vi "tcp_get_data.vi"(8 "error in":errorcluster, 10 "devs_info":T1[](array[typedef]), 11 "TCP Network Connection in":refnum<k5>) -> (0 "error out":errorcluster, 2 "data_out":u8[][](array[numeric]), 3 "TCP Network Connection out":refnum<k5>)   [LabVIEW 2021]
uses:
  typedefs/dev_full_info.ctl
  typedefs/dev_states.ctl
  typedefs/send_states.ctl
  typedefs/w5500_cmd.ctl
  typedefs/w5500_pck.ctl
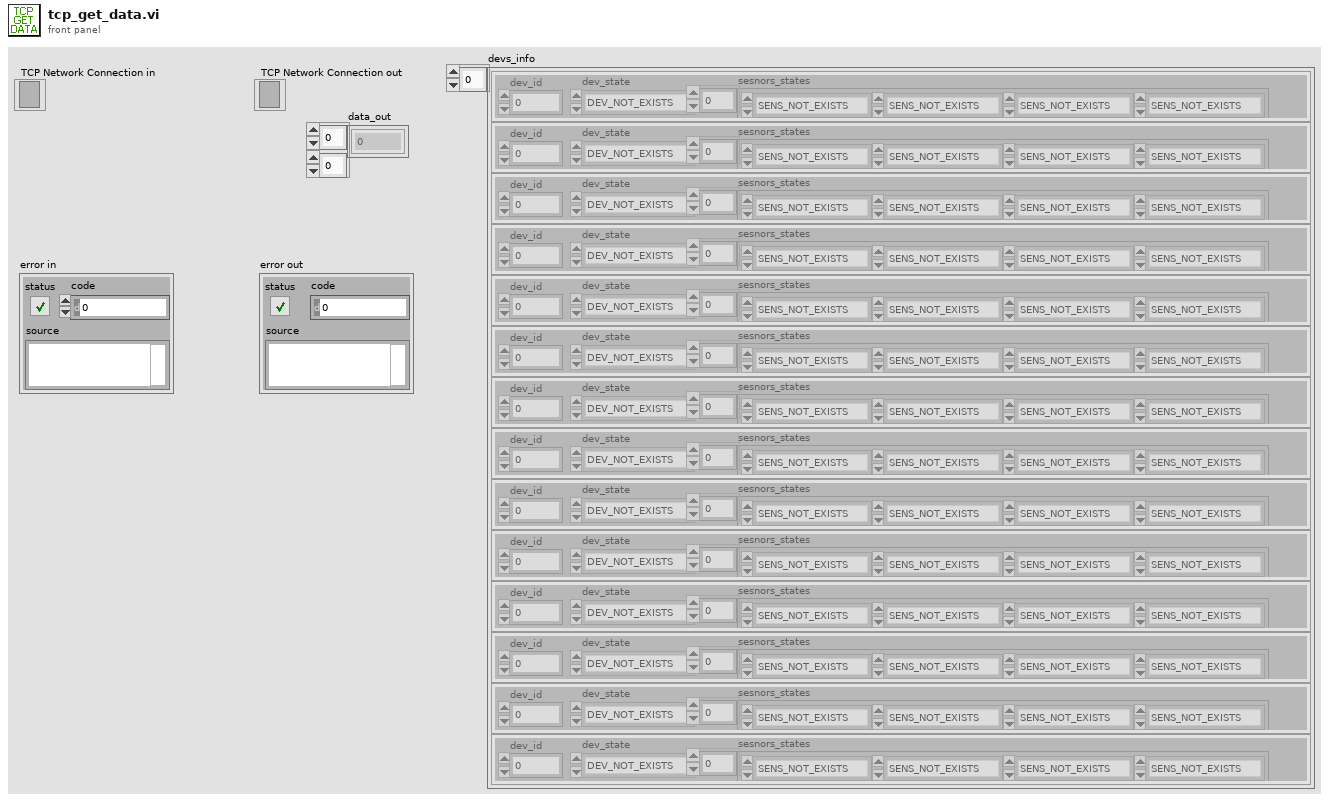
[diagram p1: front panel]
types:
  T1 = typedef "dev_full_info.ctl" = cluster{"dev_id":u32, "dev_state":T2, "sesnors_states":T3[]}
  T2 = typedef "dev_states.ctl" = enum16{"DEV_NOT_EXISTS", "DEV_EXISTS", "DEV_ERROR", "DEV_CRC_ERROR"}
  T3 = typedef "send_states.ctl" = enum16{"SENS_NOT_EXISTS", "SENS_EXISTS"}
  T4 = typedef "w5500_pck.ctl" = cluster{"cmd_type":T5, "pck_num":u32, "dev_id":u32, "data":u8[]}
  T5 = typedef "w5500_cmd.ctl" = enum32{"LAN_TRANS_START", "LAN_DATA_SZ", "LAN_CHUNK_SEND", "LAN_CHUNK_ACK", "LAN_DEVS_INFO", "LAN_DEVS_NUM", "LAN_DEVS_EXS", "LAN_DEVS_ACK", "LAN_CMD_ACK", "LAN_CMD_FIN", "LAN_SND_STAT", "LAN_REQ_STAT", "LAN_ANS_STAT", "LAN_ERR_STAT", "LAN_SETT_SET", "LAN_SETT_GET", "LAN_SETT_ACK", "LAN_SETT_ERR"}
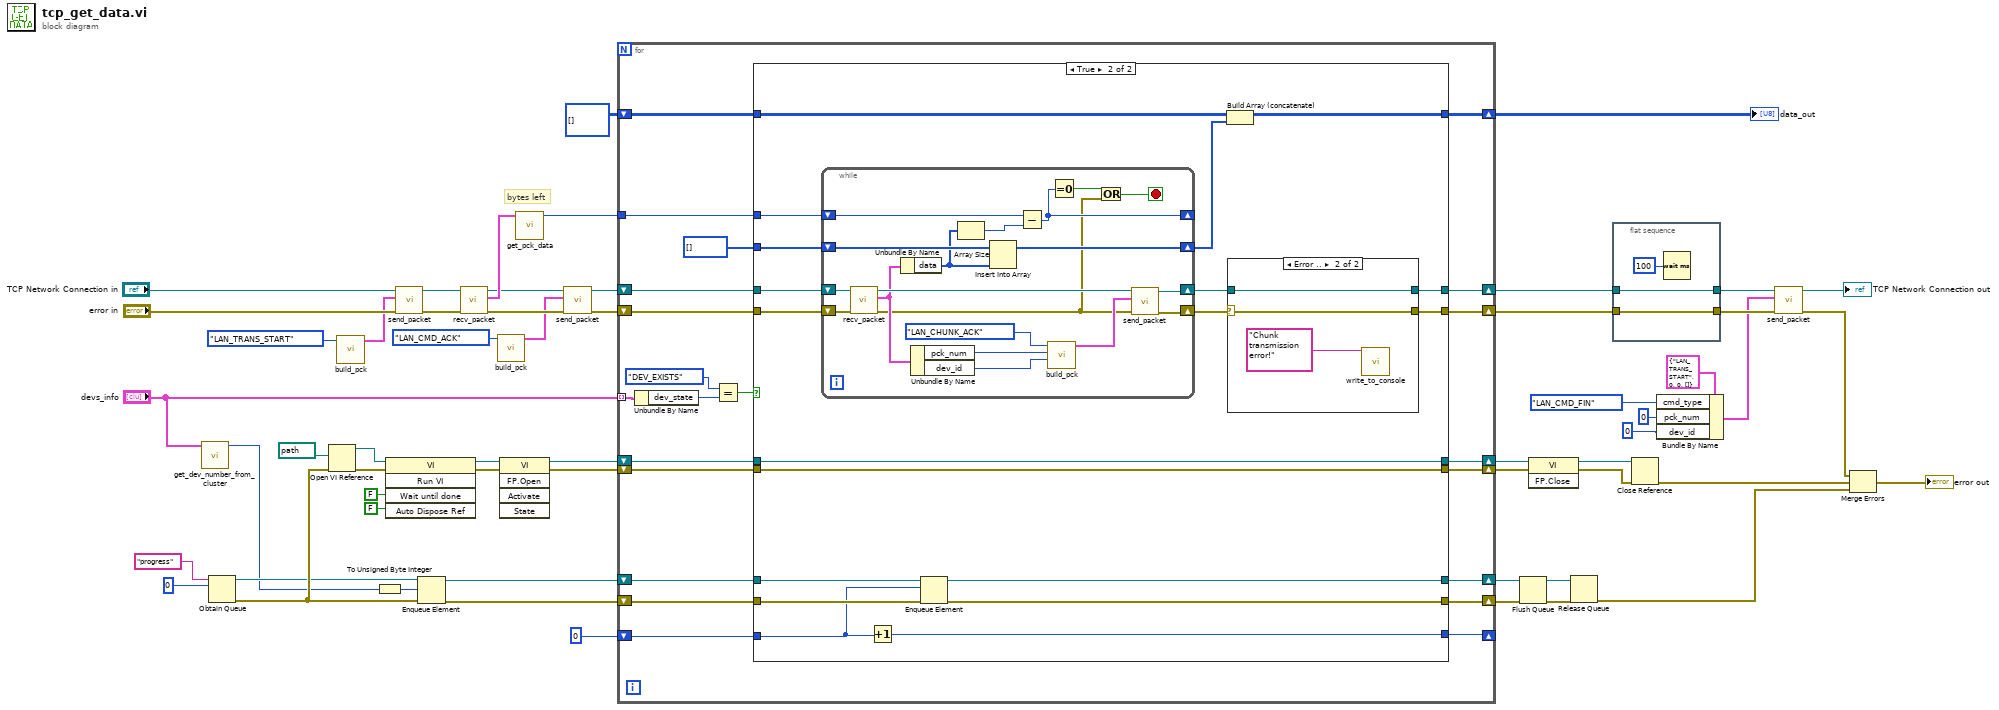
[diagram p0: block diagram]
diagram:
  # "bytes left"
  n1 = call "get_dev_number_from_cluster.vi"("devs_info"="devs_info") -> ("dev_num"=w13:u16)  [unwired: 10 in]
  n2 = Obtain Queue(name (unnamed)="progress", element data type=u8 0) -> (queue out=w20:refnum<queue>, error out=w21:errorcluster)  [unwired: 3 in, 1 out]
  n3 = Open VI Reference(vi path=path "C:/Users/Mi/YandexDisk/BigProjects/Линейки Холлов/lv2021/Users/Mi/YandexDisk/BigProjects/Линейки Холлов/labview/utils/progress_bar.vi", error in (no error)=w21) -> (vi reference=w29:refnum<vi>, error out=w28:errorcluster)  [unwired: 4 in]
  n4 = call "build_pck.vi"("cmd_type"=w5500_cmd."LAN_TRANS_START") -> ("w5500_pck"=w45:T4)  [unwired: 10 in]
  n5 = To Unsigned Byte Integer(number=w13) -> (unsigned 8bit integer=w14:u8)
  n6 = invoke class="VI" method="Run VI"(reference=w29, error in=w28, "Wait until done"=FALSE ("Wait Until Done"), "Auto Dispose Ref"=FALSE ("Auto Dispose Reference")) -> (reference out=w22:refnum<vi>, error out=w23:errorcluster)  [unwired: 1 in, 3 out]
  n7 = call "send_packet.vi"("error in (no error)"="error in", "w5500_pck in"=w45, "TCP Network Connection in"="TCP Network Connection in") -> ("error out"=w53:errorcluster, "TCP Network Connection out"=w54:refnum<k5>)  [unwired: 7 in]
  n8 = Enqueue Element(queue=w20, element=w14, error in (no error)=w21) -> (queue out=w16:refnum<queue>, error out=w17:errorcluster)  [unwired: 1 in, 1 out]
  n9 = call "recv_packet.vi"("error in (no error)"=w53, "TCP Network Connection in"=w54) -> ("error out"=w41:errorcluster, "w5500_pck"=w46:T4, "TCP Network Connection out"=w42:refnum<k5>)  [unwired: 7 in]
  n10 = call "build_pck.vi"("cmd_type"=w5500_cmd."LAN_CMD_ACK") -> ("w5500_pck"=w37:T4)  [unwired: 10 in]
  n11 = invoke class="VI" method="FP.Open"(reference=w22, error in=w23) -> (reference out=w19:refnum<vi>, error out=w18:errorcluster)  [unwired: 3 in, 3 out]
  n12 = call "get_pck_data.vi"("w5500_pck"=w46) -> ("Numeric"=w47:u32)  [unwired: 10 in]
  n13 = call "send_packet.vi"("error in (no error)"=w41, "w5500_pck in"=w37, "TCP Network Connection in"=w42) -> ("error out"=w40:errorcluster, "TCP Network Connection out"=w39:refnum<k5>)  [unwired: 7 in]
  n14 = for {
    tunnel: w47 -> [w77]
    shift-right: [w78] -> w49
    shift-left: w40 -> [w76]
    shift-right: [w79] -> w51
    shift-left: w39 -> [w75]
    tunnel: "devs_info" -> [w69] mode=indexing
    shift-right: [w71] -> w32
    shift-left: u8[][] [] -> [w72]
    shift-right: [w64] -> _
    shift-left: u8 0 -> [w65]
    shift-right: [w62] -> w8
    shift-left: w16 -> [w66]
    shift-right: [w63] -> w7
    shift-left: w17 -> [w67]
    shift-right: [w60] -> w11
    shift-left: w18 -> [w61]
    shift-right: [w58] -> w12
    shift-left: w19 -> [w59]
    n15 = Unbundle By Name(w69) -> ("dev_state"=w68:T2)
    n16 = Equal?(x=dev_states."DEV_EXISTS", y=w68) -> (x = y?=w73:bool)
    n17 = case shown="True" w73 {
      tunnel: [w87 w90] -> w79
      tunnel: [w86 w88] -> w78
      tunnel: w77 -> [_ w106]
      tunnel: w76 -> [w86 w105]
      tunnel: w75 -> [w87 w104]
      tunnel: w72 -> [w85 w103]
      tunnel: [w85 w101] -> w71
      tunnel: u8[] [] -> [_ w100]
      tunnel: w67 -> [w83 w99]
      tunnel: w66 -> [w82 w98]
      tunnel: w65 -> [w84 w97]
      tunnel: [w84 w96] -> w64
      tunnel: [w83 w95] -> w63
      tunnel: [w82 w94] -> w62
      tunnel: w61 -> [w81 w93]
      tunnel: [w81 w93] -> w60
      tunnel: w59 -> [w80 w92]
      tunnel: [w80 w92] -> w58
      frame False {
      }
      frame True {
        n18 = while {
          shift-right: [w123] -> _
          shift-left: w106 -> [w126]
          shift-right: [w120] -> w89
          shift-left: w105 -> [w130]
          shift-right: [w119] -> w91
          shift-left: w104 -> [w129]
          shift-right: [w127] -> w102
          shift-left: w100 -> [w128]
          stop <- w113 stop-if-true
          n19 = call "recv_packet.vi"("error in (no error)"=w130, "TCP Network Connection in"=w129) -> ("error out"=w112:errorcluster, "w5500_pck"=w121:T4, "TCP Network Connection out"=w122:refnum<k5>)  [unwired: 7 in]
          n20 = Unbundle By Name(w121) -> ("data"=w125:u8[])
          n21 = Unbundle By Name(w121) -> ("pck_num"=w117:u32, "dev_id"=w115:u32)
          n22 = Array Size(array=w125) -> (size(s)=w124:i32)
          n23 = Insert Into Array(array=w128, new element=w125) -> (w127:u8[])  [unwired: 1 in]
          n24 = Subtract(x=w126, y=w124) -> (x-y=w123:u32)
          n25 = call "build_pck.vi"("dev_id"=w115, "pck_num"=w117, "cmd_type"=w5500_cmd."LAN_CHUNK_ACK") -> ("w5500_pck"=w116:T4)  [unwired: 8 in]
          n26 = Equal To 0?(x=w123) -> (x = 0?=w114:bool)
          n27 = Or(x=w114, y=w112) -> (x .or. y?=w113:bool)
          n28 = call "send_packet.vi"("error in (no error)"=w112, "w5500_pck in"=w116, "TCP Network Connection in"=w122) -> ("error out"=w120:errorcluster, "TCP Network Connection out"=w119:refnum<k5>)  [unwired: 7 in]
        }
        n29 = Increment(x=w97) -> (x+1=w96:u8)
        n30 = Enqueue Element(queue=w98, element=w97, error in (no error)=w99) -> (queue out=w94:refnum<queue>, error out=w95:errorcluster)  [unwired: 1 in, 1 out]
        n31 = Build Array (concatenate)(w103, w102) -> (w101:u8[][])
        n32 = case shown="Error .." w89 {
          selector: w89 -> [w108 w111]
          tunnel: [w108 w111] -> w88
          tunnel: w91 -> [w107 w110]
          tunnel: [w107 w110] -> w90
          frame No Error {
          }
          frame Error {
            n33 = call "write_to_console.vi"("input_str"="Chunk transmission error!") -> ()  [unwired: 10 in, 1 out]
          }
        }
      }
    }
  }
  "data_out" <- w32
  n34 = Flush Queue(queue=w8, error in (no error)=w7) -> (queue out=w5:refnum<queue>, error out=w6:errorcluster)  [unwired: 1 out]
  n35 = invoke class="VI" method="FP.Close"(reference=w12, error in=w11) -> (reference out=w10:refnum<vi>, error out=w9:errorcluster)  [unwired: 1 in, 1 out]
  n36 = Release Queue(queue=w5, error in (no error)=w6) -> (error out=w3:errorcluster)  [unwired: 1 in, 2 out]
  n37 = flat-sequence {
    tunnel: w49 -> [w133]
    tunnel: [w133] -> w50
    tunnel: w51 -> [w132]
    tunnel: [w132] -> w52
    frame #0 {
      n38 = Wait (ms)(milliseconds to wait=u32 100) -> ()  [unwired: 1 out]
    }
  }
  n39 = Close Reference(reference=w10, error in (no error)=w9) -> (error out=w2:errorcluster)
  n40 = Bundle By Name(cluster=T4 {"cmd_type"=enum."LAN_TRANS_START", "pck_num"=0, "dev_id"=0, "data"=[]} ("w5500_pck"), "cmd_type"=w5500_cmd."LAN_CMD_FIN", "pck_num"=u32 0, "dev_id"=u32 0) -> (w48:T4)
  n41 = call "send_packet.vi"("error in (no error)"=w50, "w5500_pck in"=w48, "TCP Network Connection in"=w52) -> ("error out"=w1:errorcluster, "TCP Network Connection out"=→"TCP Network Connection out":refnum<k5>)  [unwired: 7 in]
  n42 = Merge Errors(w1, w2, w3) -> (→"error out":errorcluster)
